vi "Read Step Data (DC Parallel L2N Program Mode).vi"(0 "VISA resource name":refnum<visa-resource-name>, 5 "Step (1)":i32=1 min=1 max=9 format="%2_0f", 11 "error in (no error)":errorcluster) -> (4 "VISA resource name out":refnum<visa-resource-name>, 6 "Test Meter Data Output":T1 {"Timer" format="%.1f"; "Voltage (V)" format="%.1f"; "RMS Current (A)" format="%.3f"; "Power (W)" format="%.1f"}, 15 "error out":errorcluster)   [LabVIEW 2016, in "APT 300XAC Series.lvlib"]
doc: "Reads the DC mode <B>Step data</B>. \n\nIn DC Mode the output data cluster has the following data.\n\n1. Memory\n2. Step\n3. Voltage (V)\n4. Current (A)\n5. Power (W)\n5. Status"
uses:
  APT 300XAC Series.lvlib
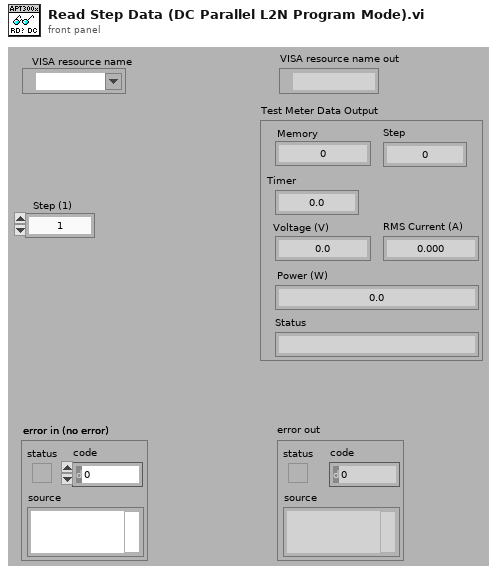
[diagram p1: front panel]
types:
  T1 = cluster{"Memory":i32, "Step":dbl, "Voltage (V)":dbl, "RMS Current (A)":dbl, "Power (W)":dbl, "Status":string, "Timer":dbl}
  T2 = cluster{"Memory":i32, "Step":dbl, "Volt":dbl, "Current":dbl, "Power":dbl, "Status":string, "Timer":dbl}
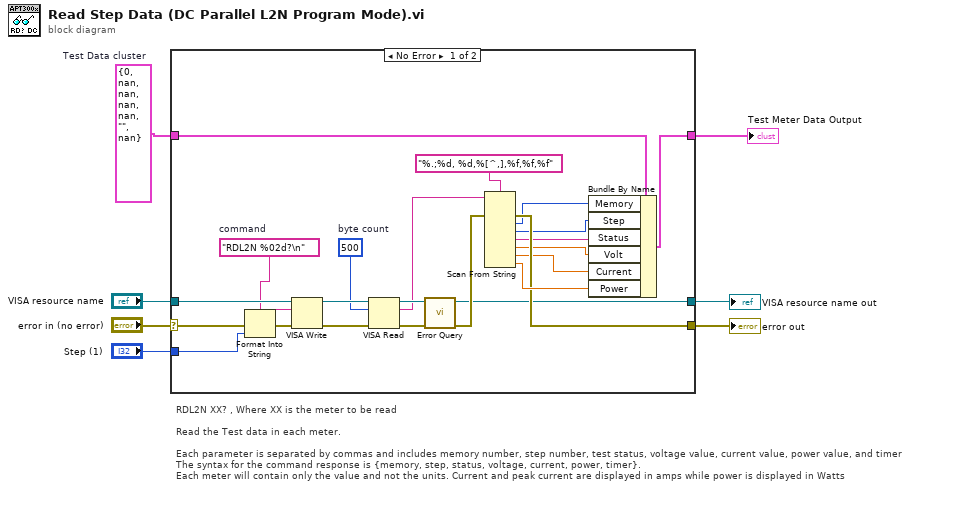
[diagram p0: block diagram]
diagram:
  w2 = T2 {"Memory"=0, "Step"=nan, "Volt"=nan, "Current"=nan, "Power"=nan, "Status"="", "Timer"=nan}  # Test Data cluster
  # "RDL2N XX? , Where XX is the meter to be read\n\nRead the Test data in each meter. \n\nEach parameter is separated by commas and includes memory number, step number, test status, voltage value, current value, power value, and timer\nThe syntax for the command response is {memory, step, status, voltage, current, power, timer}. \nEach meter will contain only the value and not the units. Current and peak current are displayed in amps while power is displayed in Watts"
  n1 = case shown="No Error" "error in (no error)" {
    selector: "error in (no error)" -> [w27 w33]
    tunnel: "VISA resource name" -> [w28 w34]
    tunnel: [w16 w34] -> w5
    tunnel: [w17 w33] -> w4
    tunnel: [w15 w32] -> w1
    tunnel: w2 -> [w14 w32]
    tunnel: "Step (1)" -> [w21 _]
    frame No Error {
      w23 = "RDL2N %02d?\n"  # command
      w29 = u32 500  # byte count
      n2 = Format Into String(format string=w23, error in=w27, w21) -> (resulting string=w22:string, error out=w24:errorcluster)  [unwired: 1 in]
      n3 = VISA Write(VISA resource name=w28, write buffer=w22, error in (no error)=w24) -> (VISA resource name out=w31:refnum<visa-resource-name>, error out=w30:errorcluster)  [unwired: 1 out]
      n4 = VISA Read(VISA resource name=w31, byte count=w29, error in (no error)=w30) -> (VISA resource name out=w26:refnum<visa-resource-name>, read buffer=w13:string, error out=w25:errorcluster)  [unwired: 1 out]
      n5 = call "Error Query.vi"("VISA resource name"=w26, "error in (no error)"=w25) -> ("VISA resource name out"=w16:refnum<visa-resource-name>, "error out"=w18:errorcluster)  [unwired: 10 in, 2 out]
      n6 = Scan From String(format string="%.;%d, %d,%[^,],%f,%f,%f", input string=w13, error in=w18) -> (error out=w17:errorcluster, output 1=w12:i32, output 2=w8:i32, output 3=w11:string, output 4=w10:dbl, output 5=w9:dbl, output 6=w19:dbl)  [unwired: 7 in, 2 out]
      n7 = Bundle By Name(cluster=w14, "Memory"=w12, "Step"=w8, "Status"=w11, "Volt"=w10, "Current"=w9, "Power"=w19) -> (w15:T2)
    }
    frame Error {
    }
  }
  "VISA resource name out" <- w5
  "error out" <- w4
  "Test Meter Data Output" <- w1
